vi "report.vi"() -> ()   [LabVIEW 2017]
uses:
  <vilib>/addons/database/Connection.llb/DB Tools Open Connec (Path).vi
  <vilib>/Utility/file.llb/Write Delimited Spreadsheet (string).vi
  <vilib>/addons/database/NI_Database_API.lvlib
  Brembo_DOCKING_2017/Source_Code/BREMBO_DOCKING_FOUR/Brembo V3.6_Thrd_m9_v7/GLobal_variable/Login Details.vi
panel:
  in  "delete":bool
  in  "Scan Barcode":bool
  out "error out":errorcluster
  in  "error in (no error)":errorcluster
  in  "FROM":timestamp format="%<%x>T"
  in  "TO":timestamp format="%<%x>T"
  out "table":string[][](table)
  out "Table header":string[](array[string])
  in  "Barcode":string
  in  "Type Wise":enum16{"Barcode Wise", "Datewise"}(ring)=enum."Datewise"
  in  "stop":bool
  in  "Export to Excel":bool
  in  "Get Report":bool
  # "REPORT"
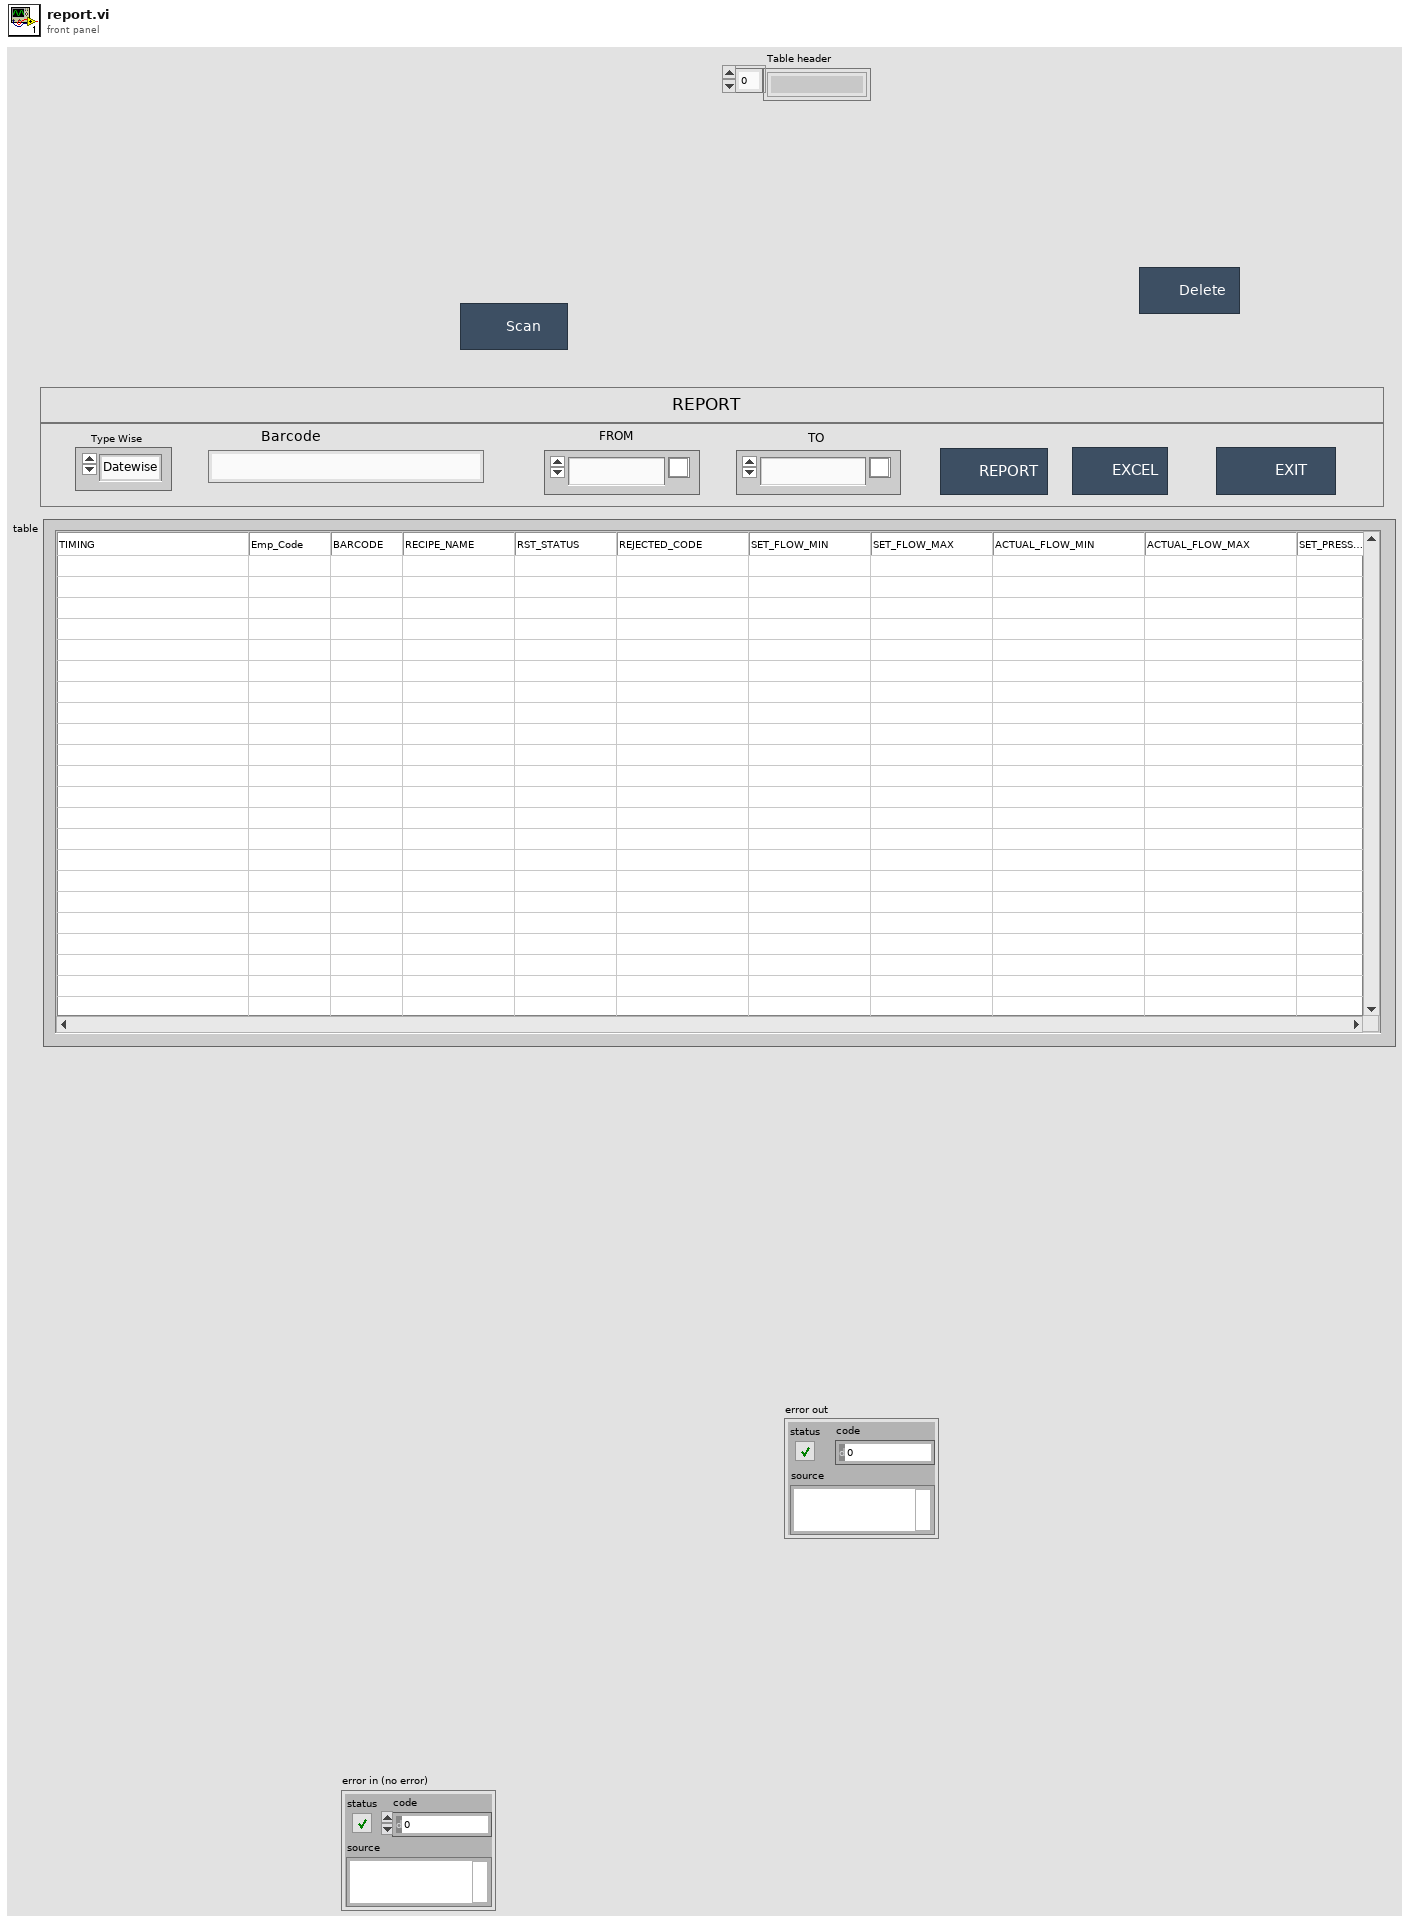
[diagram p1: front panel]
types:
  T1 = typedef "LVDateTimeRec.ctl" = cluster{"fractional second":dbl, "second":i32, "minute":i32, "hour":i32, "day of month":i32, "month":i32, "year":i32, "day of week":i32, "day of year":i32, "DST":i32}
  T2 = typedef "NI_Database_API.lvlib/Conn ObjectReference.ctl" = refnum<k1>
  T3 = enum16{"open", "replace", "create", "open or create", "replace or create", "replace or create with confirmation"}
  T4 = enum32{"invalid app kind", "Development System", "Run Time System", "Student Edition", "Embedded LabVIEW", "Evaluation", "Custom"}
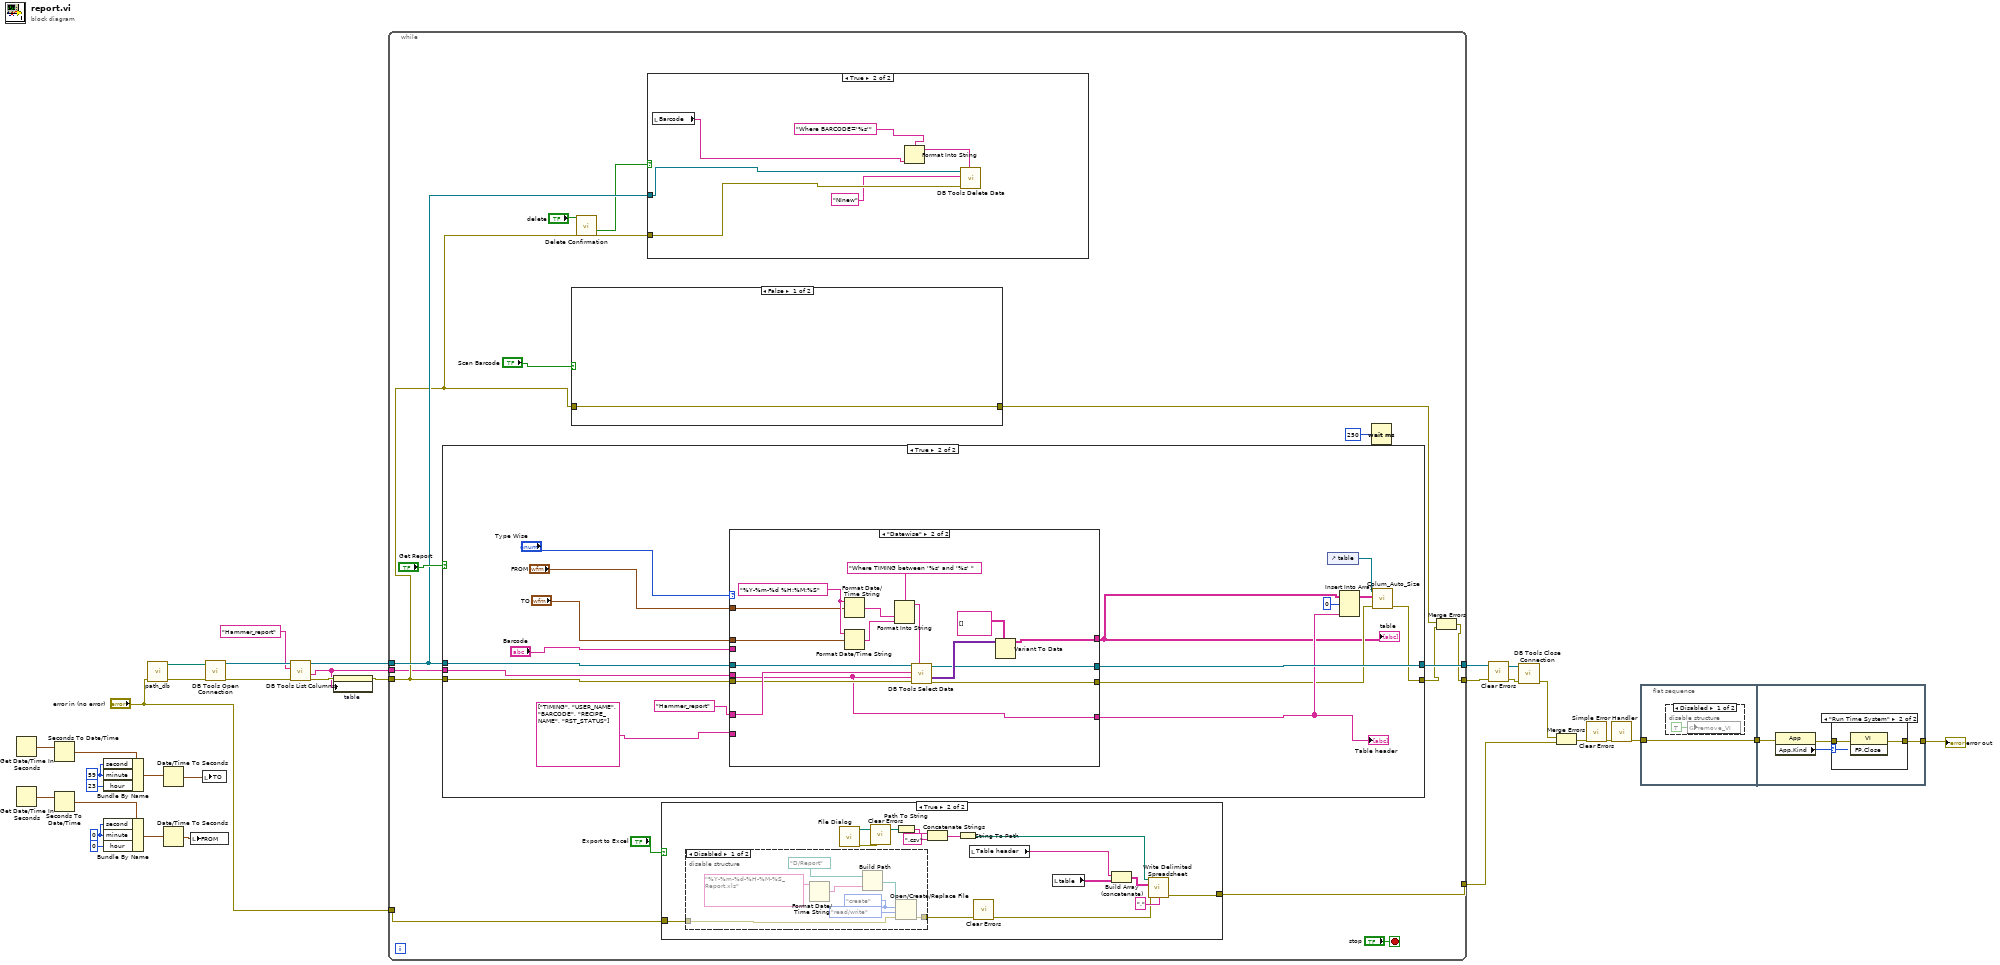
[diagram p0: block diagram]
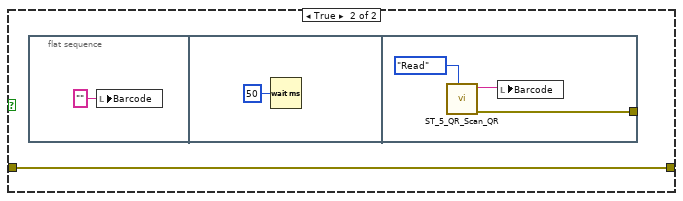
[diagram p5: hidden frame]
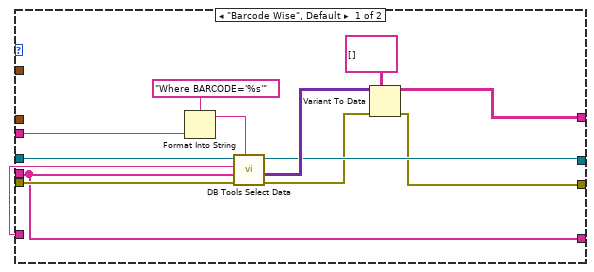
[diagram p9: hidden frame]
diagram:
  w26 = 0 ("minute")
  w27 = 59 ("minute")
  n1 = Get Date/Time In Seconds() -> (seconds since 1Jan1904=w29:timestamp)
  n2 = Get Date/Time In Seconds() -> (seconds since 1Jan1904=w24:timestamp)
  n3 = Seconds To Date/Time(time stamp (now)=w29) -> (date time rec=w30:T1)  [unwired: 1 in]
  n4 = Seconds To Date/Time(time stamp (now)=w24) -> (date time rec=w23:T1)  [unwired: 1 in]
  n5 = Bundle By Name(cluster=w30, "second"=w27, "minute"=w27, "hour"=23) -> (w31:T1)
  n6 = Bundle By Name(cluster=w23, "second"=w26, "minute"=w26, "hour"=0) -> (w22:T1)
  n7 = call "path_db.vi"("error in"="error in (no error)") -> ("error out"=w11:errorcluster, "resulting string"=w12:path)  [unwired: 9 in]
  n8 = Date/Time To Seconds(2:w31) -> (0:w20:timestamp)  [unwired: 1 in]
  n9 = Date/Time To Seconds(2:w22) -> (0:w21:timestamp)  [unwired: 1 in]
  n10 = local write "FROM"(w21) -> ()
  n11 = local write "TO"(w20) -> ()
  n12 = call-poly <vilib>:"DB Tools Open Connection.vi"("error in (no error)"=w11, "connection information"=w12) -> ("error out"=w7:errorcluster, "connection reference"=w6:T2)  [unwired: 6 in]
  n13 = call <vilib>:"DB Tools List Columns.vi"("error in (no error)"=w7, "table"="Hammer_report", "connection reference"=w6) -> ("error out"=w3:errorcluster, "columns"=w1:string[], "connection reference out"=w5:T2)  [unwired: 1 in, 1 out]
  n14 = property on="table" class="Tbl (strict)"(error in=w3, "Column Headers[]"=w1) -> (error out=w2:errorcluster)  [unwired: 1 in, 1 out]
  n15 = while {
    tunnel: w5 -> [w38]
    tunnel: w2 -> [w37]
    tunnel: [w49] -> w19
    tunnel: [w39] -> w9
    tunnel: "error in (no error)" -> [w47]
    tunnel: [w46] -> w17
    tunnel: w1 -> [w33]
    stop <- "stop" stop-if-true
    n16 = case shown="True" "Get Report" {
      tunnel: w38 -> [w87 w103]
      tunnel: w37 -> [w86 w102]
      tunnel: [w87 w101] -> w49
      tunnel: [w86 w95] -> w40
      tunnel: w33 -> [_ w88]
      frame False {
      }
      frame True {
        n17 = case shown="\"Datewise\"" "Type Wise" {
          tunnel: w103 -> [w117 w133]
          tunnel: w102 -> [w116 w119]
          tunnel: string[] ["TIMING", "USER_NAME", "BARCODE", "RECIPE_NAME", "RST_STATUS"] -> [_ _]
          tunnel: "Hammer_report" ("table") -> [w111 w130]
          tunnel: [w110 w129] -> w101
          tunnel: [w108 w128] -> w91
          tunnel: [w107 w122] -> w89
          tunnel: [w105 w118] -> w97
          tunnel: "Barcode" -> [w106 _]
          tunnel: "FROM" -> [_ w121]
          tunnel: "TO" -> [_ w120]
          tunnel: w88 -> [w105 w118]
          frame "Barcode Wise", Default {
            n18 = Format Into String(format string="Where BARCODE='%s'", w106) -> (resulting string=w114:string)  [unwired: 2 in, 1 out]
            n19 = call <vilib>:"DB Tools Select Data.vi"("condition"=w114, "error in (no error)"=w116, "columns"=w105, "table"=w111, "connection reference"=w117) -> ("error out"=w109:errorcluster, "data"=w113:variant[][], "connection reference out"=w110:T2)  [unwired: 1 in]
            n20 = Variant To Data(error in=w109, type=string[][] [], Variant=w113) -> (data=w107:string[][], error out=w108:errorcluster)
          }
          frame "Datewise" {
            w124 = "%Y-%m-%d %H:%M:%S" ("time format string (%c)")
            n21 = Format Date/Time String(time format string (%c)=w124, seconds (now)=w120) -> (date/time string=w125:string)  [unwired: 1 in]
            n22 = Format Date/Time String(time format string (%c)=w124, seconds (now)=w121) -> (date/time string=w126:string)  [unwired: 1 in]
            n23 = Format Into String(format string="Where TIMING between '%s' and '%s' ", w126, w125) -> (resulting string=w127:string)  [unwired: 2 in, 1 out]
            n24 = call <vilib>:"DB Tools Select Data.vi"("condition"=w127, "error in (no error)"=w119, "columns"=w118, "table"=w130, "connection reference"=w133) -> ("error out"=w128:errorcluster, "data"=w132:variant[][], "connection reference out"=w129:T2)  [unwired: 1 in]
            n25 = Variant To Data(type=string[][] [], Variant=w132) -> (data=w122:string[][])  [unwired: 1 in, 1 out]
          }
        }
        "table" <- w89
        "Table header" <- w97
        n26 = control-ref of="table"() -> (w94:refnum<vi>)
        n27 = Insert Into Array(array=w89, index (row)=0, new element=w97) -> (w93:string[][])  [unwired: 1 in]
        n28 = call "Colum_Auto_Size.vi"("error in (no error)"=w91, "Table With header"=w93, "Table reference"=w94) -> ("error out"=w95:errorcluster)  [unwired: 8 in]
      }
    }
    n29 = case shown="False" "Scan Barcode" {
      tunnel: w37 -> [w56 w57]
      tunnel: [w56 w57] -> w41
      frame False {
      }
      frame True {
        n30 = flat-sequence {
          tunnel: [w60] -> _
          frame #0 {
            n31 = local write "Barcode"("" ("Barcode")) -> ()
          }
          frame #1 {
            n32 = Wait (ms)(milliseconds to wait=u32 50) -> ()  [unwired: 1 out]
          }
          frame #2 {
            n33 = call "ST_5_QR_Scan_QR.vi"("Enum"=enum16{"Read", "Write"}."Read") -> ("error out"=w60:errorcluster, "LB QR ST 5"=w62:string)  [unwired: 9 in]
            n34 = local write "Barcode"(w62) -> ()
          }
        }
      }
    }
    n35 = call "Delete Confirmation"("Enable"="delete", "error in (no error)"=w37) -> ("OK"=w34:bool, "error out"=w36:errorcluster)  [unwired: 16 in]
    n36 = case shown="True" w34 {
      tunnel: w38 -> [_ w55]
      tunnel: w36 -> [_ w54]
      frame False {
      }
      frame True {
        n37 = local read "Barcode"() -> (w53:string)
        n38 = Format Into String(format string="Where BARCODE='%s'", w53) -> (resulting string=w52:string)  [unwired: 2 in, 1 out]
        n39 = call <vilib>:"DB Tools Delete Data.vi"("condition"=w52, "error in (no error)"=w54, "table"="NInew", "connection reference"=w55) -> ()  [unwired: 6 in, 2 out]
      }
    }
    n40 = case shown="True" "Export to Excel" {
      tunnel: w47 -> [w63 w77]
      tunnel: [w63 w76] -> w46
      frame False {
      }
      frame True {
        n41 = disable-structure shown="Disabled" {
          disable-tunnel: w77 -> [w81 w85]
          disable-tunnel: [w80 w85] -> w65
          frame Disabled {
            w78 = enum16{"read/write", "read-only", "write-only"}."read/write" ("access (0:read/write)")
            w78 = T3."create" ("operation (0:open)")
            n42 = Format Date/Time String(time format string (%c)="%Y-%m-%d-%H-%M-%S_Report.xls") -> (date/time string=w84:string)  [unwired: 2 in]
            n43 = Build Path(base path=path "D:/Report", name or relative path=w84) -> (appended path=w82:path)
            n44 = Open/Create/Replace File(file path (use dialog)=w82, error in=w81, operation (0:open)=w78, access (0:read/write)=w78) -> (error out=w80:errorcluster)  [unwired: 2 in, 2 out]
          }
          frame Enabled {
          }
        }
        n45 = call "File Dialog"() -> ("selected path"=w70:path, "error out"=w71:errorcluster)  [unwired: 12 in, 2 out]
        n46 = call <vilib>:"Clear Errors.vi"("error in (no error)"=w71) -> ()  [unwired: 5 in, 2 out]
        n47 = Path To String(path=w70) -> (string=w69:string)
        n48 = Concatenate Strings(w69, ".csv" ("string")) -> (w67:string)
        n49 = String To Path(string=w67) -> (path=w66:path)
        n50 = local read "Table header"() -> (w73:string[])
        n51 = call <vilib>:"Clear Errors.vi"("error in (no error)"=w65) -> ("error out"=w64:errorcluster)  [unwired: 5 in, 1 out]
        n52 = local read "table"() -> (w74:string[][])
        n53 = Build Array (concatenate)(w73, w74) -> (w75:string[][])
        n54 = call-poly <vilib>:"Write Delimited Spreadsheet.vi"("file path (dialog if empty)"=w66, "2D data"=w75, "error in (no error)"=w64, "delimiter (\\t)"="," ("delimiter (\\t)")) -> ("error out"=w76:errorcluster)  [unwired: 10 in, 1 out]
      }
    }
    n55 = Wait (ms)(milliseconds to wait=u32 250) -> ()  [unwired: 1 out]
    n56 = Merge Errors(w41, w40) -> (w39:errorcluster)
  }
  n57 = call <vilib>:"Clear Errors.vi"("error in (no error)"=w9) -> ("error out"=w8:errorcluster)  [unwired: 5 in, 1 out]
  n58 = call <vilib>:"DB Tools Close Connection.vi"("error in (no error)"=w8, "connection reference"=w19) -> ("error out"=w18:errorcluster)  [unwired: 5 in]
  n59 = Merge Errors(w18, w17) -> (w16:errorcluster)
  n60 = call <vilib>:"Clear Errors.vi"("error in (no error)"=w16) -> ("error out"=w15:errorcluster)  [unwired: 5 in, 1 out]
  n61 = call <vilib>:"Simple Error Handler.vi"("error in (no error)"=w15) -> ("error out"=w14:errorcluster)  [unwired: 4 in, 4 out]
  n62 = flat-sequence {
    tunnel: w14 -> [w134]
    tunnel: [w134] -> w32
    tunnel: w32 -> [w137]
    tunnel: [w136] -> w13
    frame #0 {
      n63 = disable-structure shown="Disabled" {
        frame Disabled {
          n64 = global write "Login Details.vi" "remove_VI"(TRUE ("remove_VI")) -> ()
        }
        frame Enabled {
        }
      }
    }
    frame #1 {
      n65 = property class="App"(error in=w137) -> (error out=w138:errorcluster, "App.Kind"=w139:T4)  [unwired: 1 in, 1 out]
      n66 = case shown="\"Run Time System\"" w139 {
        tunnel: w138 -> [w140 w142]
        tunnel: [w140 w141] -> w136
        frame Default {
        }
        frame "Run Time System" {
          n67 = invoke class="VI" method="FP.Close"(error in=w142) -> (error out=w141:errorcluster)  [unwired: 2 in, 2 out]
        }
      }
    }
  }
  "error out" <- w13
